vi "Configure Marker State.vi"(7 "Marker On":bool, 8 "error in (no error)":errorcluster, 10 "Marker Number":u8=1, 11 "VNA-PNA in":refnum<class "VNA-PNA.lvclass">) -> (0 "error out":errorcluster, 3 "VNA-PNA out":refnum<class "VNA-PNA.lvclass">)   [LabVIEW 2020, in "VNA-PNA.lvclass"]
doc: "Configure the marker state.\nThe marker is on the active trace."
uses:
  VNA-PNA.lvclass
  C:/Sandbox/RF Bench/Source Code/WiSpry Test Framework/Instruments/Instrument.lvclass
  Instrument.lvclass/Instrument.ctl
  Instrument.lvclass
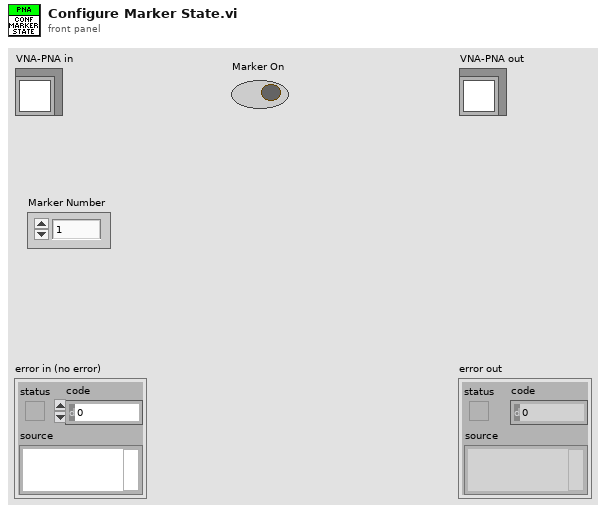
[diagram p1: front panel]
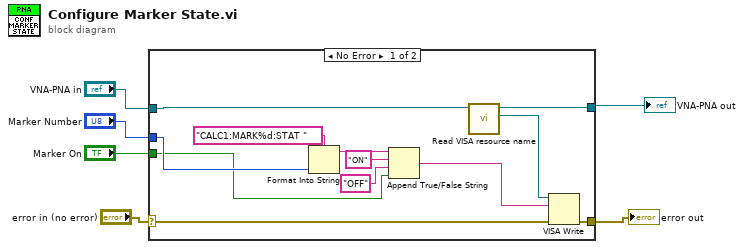
[diagram p0: block diagram]
diagram:
  n1 = case shown="No Error" "error in (no error)" {
    selector: "error in (no error)" -> [w11 w19]
    tunnel: "VNA-PNA in" -> [w12 w20]
    tunnel: "Marker Number" -> [w17 _]
    tunnel: "Marker On" -> [w13 _]
    tunnel: [w8 w20] -> w1
    tunnel: [w7 w19] -> w2
    frame No Error {
      n2 = Format Into String(format string="CALC1:MARK%d:STAT ", w17) -> (resulting string=w16:string)  [unwired: 2 in, 1 out]
      n3 = Append True/False String(1:w13, 2:"OFF" ("false string"), 3:"ON" ("true string"), 4:w16) -> (0:w10:string)
      n4 = call "Read VISA resource name.vi"("Instrument in"=w12) -> ("VISA resource name"=w9:refnum<visa-resource-name>, "Instrument out"=w8:refnum<class "VNA-PNA.lvclass">)  [unwired: 9 in]
      n5 = VISA Write(VISA resource name=w9, write buffer=w10, error in (no error)=w11) -> (error out=w7:errorcluster)  [unwired: 2 out]
    }
    frame Error {
    }
  }
  "error out" <- w2
  "VNA-PNA out" <- w1
